vi "Cleanup.vi"(8 "error in (no error)":errorcluster, 11 "Node in":refnum<class "bt_Decorator.lvclass">) -> (0 "error out":errorcluster, 3 "Node out":refnum<class "bt_Decorator.lvclass">)   [LabVIEW 2021, in "BT.lvlib" / "bt_Decorator.lvclass"]
uses:
  bt_Decorator.lvclass
  bt_Decorator.lvclass/bt_Decorator.ctl
  abs_Node/bt_Node.lvclass
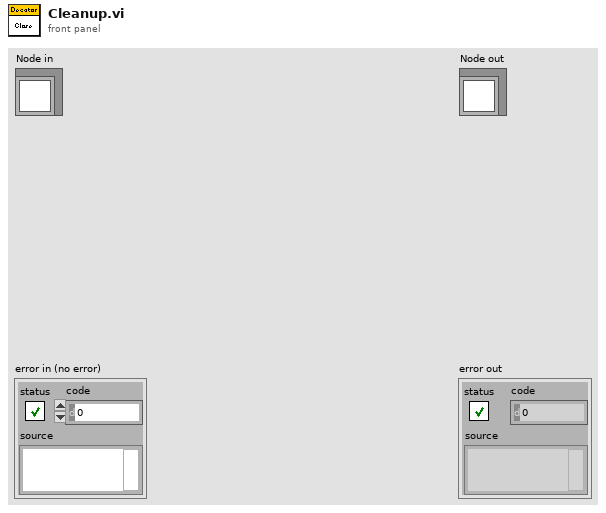
[diagram p1: front panel]
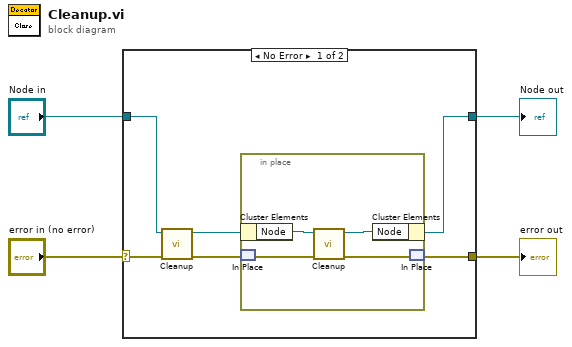
[diagram p0: block diagram]
diagram:
  n1 = case shown="No Error" "error in (no error)" {
    selector: "error in (no error)" -> [w10 w15]
    tunnel: "Node in" -> [w9 w16]
    tunnel: [w7 w16] -> w1
    tunnel: [w5 w15] -> w3
    frame No Error {
      n2 = call-parent "Cleanup.vi"("error in (no error)"=w10, "Node in"=w9) -> ("error out"=w6:errorcluster, "Node out"=w8:refnum<class "bt_Decorator.lvclass">)  [unwired: 8 in]
      n3 = in-place {
        n4 = in-place-cluster #1(w8) -> ("Node"=w14:refnum<class "bt_Node.lvclass">)
        n5 = in-place-match #2(w6) -> (w12:errorcluster)
        n6 = call-dynamic "Cleanup.vi"("error in (no error)"=w12, "Node in"=w14) -> ("error out"=w11:errorcluster, "Node out"=w13:refnum<class "bt_Node.lvclass">)  [unwired: 8 in]
        n7 = in-place-cluster #1("Node"=w13) -> (w7:refnum<class "bt_Decorator.lvclass">)
        n8 = in-place-match #2(w11) -> (w5:errorcluster)
      }
    }
    frame Error {
    }
  }
  "error out" <- w3
  "Node out" <- w1
